vi "IncludeProjectLibrary.vi"(7 "Include Sub Libraries (T)":bool=TRUE, 8 "error in (no error)":errorcluster, 10 "Path":path, 11 "Whitelist in":refnum<class "Whitelist.lvclass">) -> (0 "error out":errorcluster, 3 "Whitelist out":refnum<class "Whitelist.lvclass">)   [LabVIEW 2017, in "Whitelist.lvclass"]
doc: "Includes files from a project library in the whitelist. Includes sub libraries if <B>Include Sub Libraries</B> is enabled (default)."
uses:
  Whitelist.lvclass
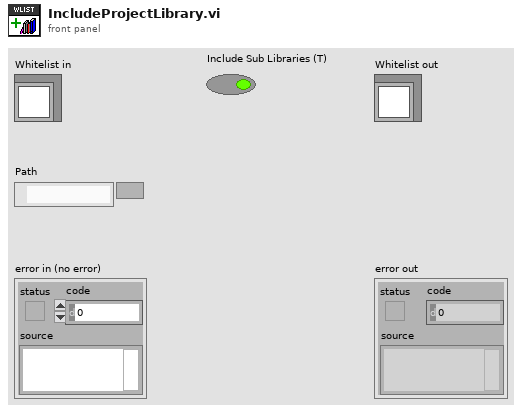
[diagram p1: front panel]
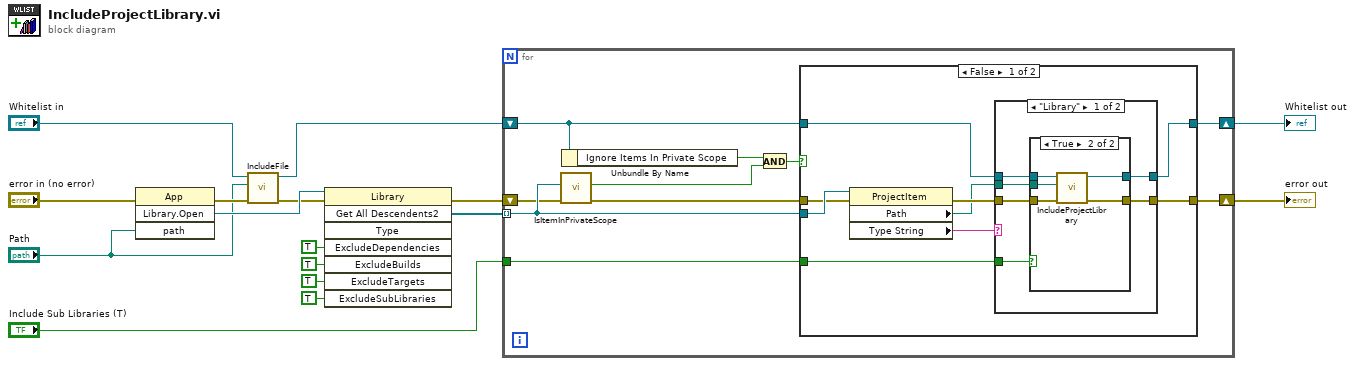
[diagram p0: block diagram]
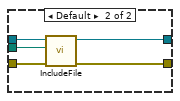
[diagram p3: hidden frame]
diagram:
  n1 = invoke class="App" method="Library.Open"(error in="error in (no error)", "path"="Path") -> (error out=w5:errorcluster, "Open Library"=w15:refnum<vi>)  [unwired: 2 in, 2 out]
  n2 = call "IncludeFile.vi"("error in (no error)"=w5, "Path"="Path", "Whitelist in"="Whitelist in") -> ("error out"=w4:errorcluster, "Whitelist out"=w1:refnum<class "Whitelist.lvclass">)  [unwired: 7 in]
  n3 = invoke class="Library" method="Get All Descendents2"(reference=w15, error in=w4, "ExcludeDependencies"=TRUE, "ExcludeBuilds"=TRUE, "ExcludeTargets"=TRUE, "ExcludeSubLibraries"=TRUE) -> (error out=w11:errorcluster, "Get All Descendents2"=w8:refnum<vi>[])  [unwired: 2 in, 6 out]
  n4 = for {
    shift-right: [w26] -> w10
    shift-left: w11 -> [w23]
    shift-right: [w25] -> w9
    shift-left: w1 -> [w21]
    tunnel: w8 -> [w24] mode=indexing
    tunnel: "Include Sub Libraries (T)" -> [w17]
    n5 = call "IsItemInPrivateScope.vi"("error in (no error)"=w23, "Item"=w24) -> ("error out"=w22:errorcluster, "Is Private?"=w19:bool)  [unwired: 8 in]
    n6 = Unbundle By Name(w21) -> ("Ignore Items In Private Scope"=w20:bool)
    n7 = And(x=w20, y=w19) -> (x .and. y?=w18:bool)
    n8 = case shown="False" w18 {
      tunnel: [w35 w54] -> w26
      tunnel: [w34 w55] -> w25
      tunnel: w24 -> [w31 _]
      tunnel: w22 -> [w30 w54]
      tunnel: w21 -> [w29 w55]
      tunnel: w17 -> [w27 _]
      frame False {
        n9 = property class="ProjectItem"(reference=w31, error in=w30) -> (error out=w33:errorcluster, "Path"=w32:path, "Type String"=w28:string)  [unwired: 1 out]
        n10 = case shown="\"Library\"" w28 {
          tunnel: [w40 w53] -> w35
          tunnel: [w38 w52] -> w34
          tunnel: w33 -> [w41 w51]
          tunnel: w32 -> [w37 w50]
          tunnel: w29 -> [w39 w49]
          tunnel: w27 -> [w36 _]
          frame "Library" {
            n11 = case shown="True" w36 {
              tunnel: w41 -> [w42 w48]
              tunnel: [w42 w47] -> w40
              tunnel: w39 -> [w43 w46]
              tunnel: [w43 w45] -> w38
              tunnel: w37 -> [_ w44]
              frame False {
              }
              frame True {
                n12 = call "IncludeProjectLibrary.vi"("error in (no error)"=w48, "Path"=w44, "Whitelist in"=w46) -> ("error out"=w47:errorcluster, "Whitelist out"=w45:refnum<class "Whitelist.lvclass">)  [unwired: 7 in]
              }
            }
          }
          frame Default {
            n13 = call "IncludeFile.vi"("error in (no error)"=w51, "Path"=w50, "Whitelist in"=w49) -> ("error out"=w53:errorcluster, "Whitelist out"=w52:refnum<class "Whitelist.lvclass">)  [unwired: 7 in]
          }
        }
      }
      frame True {
      }
    }
  }
  "error out" <- w10
  "Whitelist out" <- w9
